vi "cDAQ Barometric Pressure Convert AI Volt to Measurement.vi"(11 "AI Voltage":T1) -> (3 "Mean measurement (in. Hg)":dbl)   [LabVIEW 2014]
doc: "Converts AI voltage measurement to barometric pressure reading"
uses:
  Type Definitions/cDAQ Instrument Sensor.ctl
panel:
  in  "B":dbl=20.0
  in  "M":dbl=1.5
  out "Std dev measurement":dbl
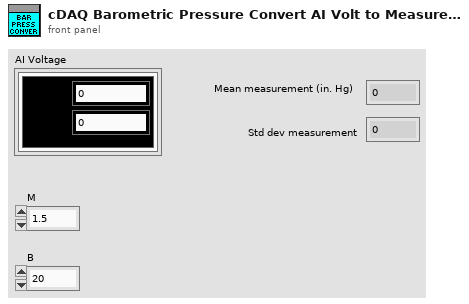
[diagram p1: front panel]
types:
  T1 = typedef "cDAQ Instrument Sensor.ctl" = cluster{"Mean":dbl, " Std":dbl, "Color Box":u32}
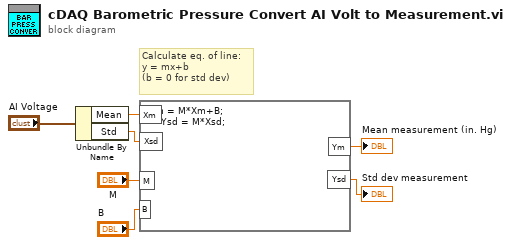
[diagram p0: block diagram]
diagram:
  # "Calculate eq. of line: \ny = mx+b \n(b = 0 for std dev)"
  n1 = Unbundle By Name("AI Voltage") -> ("Mean"=w6:dbl, "Std"=w4:dbl)
  n2 = formula code="Ym = M*Xm+B;\n    Ysd = M*Xsd;"("Xm"=w6, "Xsd"=w4, "M"="M", "B"="B") -> ("Ym"=→"Mean measurement (in. Hg)":dbl, "Ysd"=→"Std dev measurement":dbl)
